vi "Get Project MyComputer.vi"(8 "error in":errorcluster) -> (0 "error out":errorcluster, 3 "My Computer":refnum<vi>)   [LabVIEW 2021, in "Missing in Project.lvclass"]
doc: "Returns the MyComputer reference to the project."
uses:
  Missing in Project.lvclass
panel:
  out "project path":path
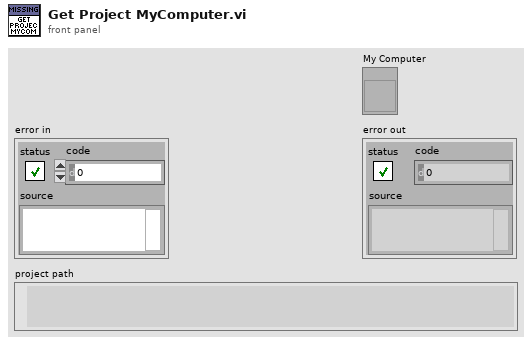
[diagram p1: front panel]
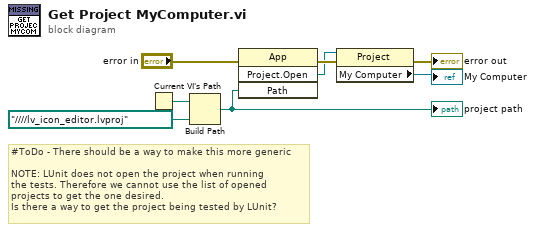
[diagram p0: block diagram]
diagram:
  # "#ToDo - There should be a way to make this more generic\n\nNOTE: LUnit does not open the project when running\nthe tests. Therefore we cannot use the list of opened\nprojects to get the one desired.\nIs there a way to get the project being tested by LUnit?"
  n1 = Current VI's Path() -> (path=w4:path)
  n2 = Build Path(base path=w4, name or relative path=path "../../../../lv_icon_editor.lvproj") -> (appended path=w2:path)
  "project path" <- w2
  n3 = invoke class="App" method="Project.Open"(error in="error in", "Path"=w2) -> (error out=w8:errorcluster, "Project:Open"=w3:refnum<vi>)  [unwired: 2 in, 2 out]
  n4 = property class="Project"(reference=w3, error in=w8) -> (error out=→"error out":errorcluster, "My Computer"=→"My Computer":refnum<vi>)  [unwired: 1 out]
